vi "Error Query.vi"(8 "error in (no error)":errorcluster, 11 "VISA resource name":refnum<visa-resource-name>) -> (0 "error out":errorcluster, 1 "Error Message":string, 2 "Error Code (00)":i32, 3 "VISA resource name out":refnum<visa-resource-name>)   [LabVIEW 2015, in "Fluke 28x Series.lvlib"]
doc: "Queries the instrument for any errors in the instrument's error queue. It will continue to read errors until all errors have been read from the instrument. Any errors will be returned in the <B>error out</B> control.\n\n<B>Note:</B>\nThis VI is called automatically by most driver VIs so it is not usually necessary to call this in an application."
uses:
  <instrlib>/Fluke 28x Series/Fluke 28x Series.lvlib
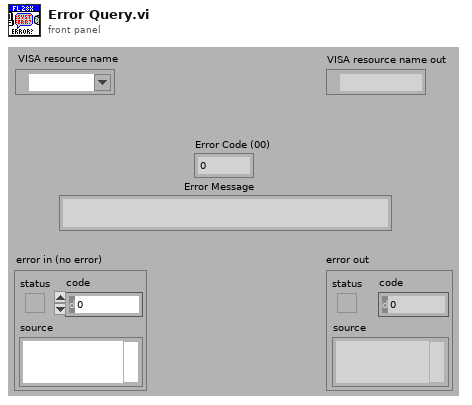
[diagram p1: front panel]
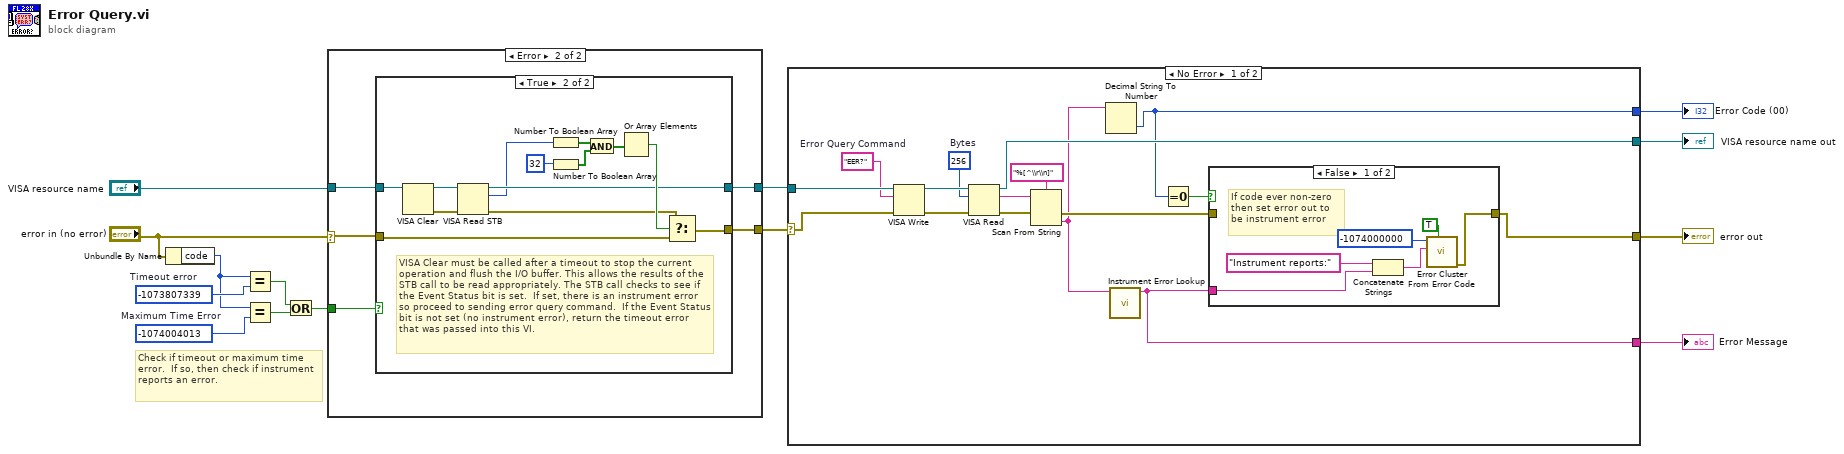
[diagram p0: block diagram]
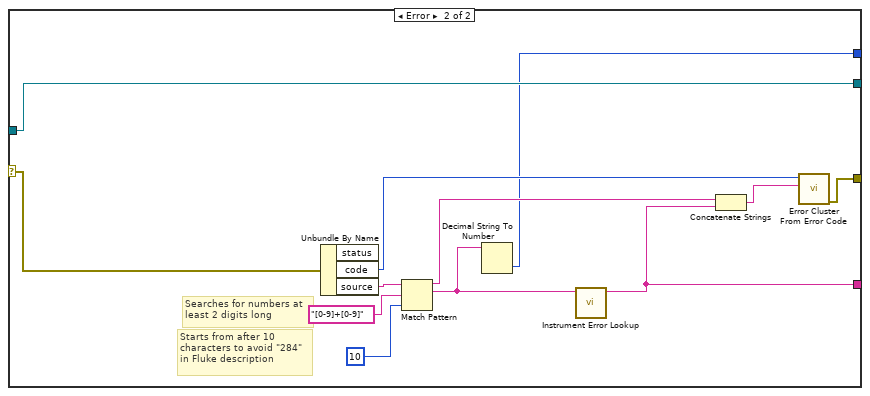
[diagram p5: hidden frame]
diagram:
  w6 = -1074004013  # Maximum Time Error
  w8 = -1073807339  # Timeout error
  # "Check if timeout or maximum time error.  If so, then check if instrument reports an error."
  n1 = Unbundle By Name("error in (no error)") -> ("code"=w7:i32)
  n2 = Equal?(x=w7, y=w8) -> (x = y?=w4:bool)
  n3 = Equal?(x=w7, y=w6) -> (x = y?=w5:bool)
  n4 = Or(x=w4, y=w5) -> (x .or. y?=w3:bool)
  n5 = case shown="Error" "error in (no error)" {
    selector: "error in (no error)" -> [w15 w19]
    tunnel: "VISA resource name" -> [w16 w21]
    tunnel: [w16 w20] -> w10
    tunnel: [w15 w18] -> w11
    tunnel: w3 -> [_ w17]
    frame No Error {
    }
    frame Error {
      n6 = case shown="True" w17 {
        tunnel: w21 -> [w23 w29]
        tunnel: [w23 w26] -> w20
        tunnel: w19 -> [w22 w32]
        tunnel: [w22 w31] -> w18
        frame False {
          # "Error code not a timeout, so best to pass on to user."
        }
        frame True {
          # "VISA Clear must be called after a timeout to stop the current operation and flush the I/O buffer. This allows the results of the  STB call to be read appropriately. The STB call checks to see if the Event Status bit is set.  If set, there is an instrument error so proceed to sending error query command.  If the Event Status bit is not set (no instrument error), return the timeout error that was passed into this VI."
          n7 = VISA Clear(VISA resource name=w29) -> (VISA resource name out=w28:refnum<visa-resource-name>, error out=w27:errorcluster)  [unwired: 1 in]
          n8 = VISA Read STB(8:w27, 11:w28) -> (0:w25:errorcluster, 2:w24:u16, 3:w26:refnum<visa-resource-name>)
          n9 = Number To Boolean Array(number=w24) -> (Boolean array=w33:bool[])
          n10 = Number To Boolean Array(number=32) -> (Boolean array=w35:bool[])
          n11 = And(x=w33, y=w35) -> (x .and. y?=w34:bool[])
          n12 = Or Array Elements(Boolean array=w34) -> (logical OR=w30:bool)
          n13 = Select(t=w25, s=w30, f=w32) -> (s? t:f=w31:errorcluster)
        }
      }
    }
  }
  n14 = case shown="No Error" w11 {
    selector: w11 -> [w50 w67]
    tunnel: [w52 w71] -> w14
    tunnel: w10 -> [w51 w71]
    tunnel: [w37 w64] -> w13
    tunnel: [w42 w62] -> w12
    tunnel: [w40 w60] -> w2
    frame No Error {
      w43 = "EER?"  # Error Query Command
      w48 = u32 256  # Bytes
      n15 = VISA Write(VISA resource name=w51, write buffer=w43, error in (no error)=w50) -> (VISA resource name out=w49:refnum<visa-resource-name>, error out=w47:errorcluster)  [unwired: 1 out]
      n16 = VISA Read(VISA resource name=w49, byte count=w48, error in (no error)=w47) -> (VISA resource name out=w52:refnum<visa-resource-name>, read buffer=w45:string, error out=w44:errorcluster)  [unwired: 1 out]
      n17 = Scan From String(format string="%[^\\r\\n]", input string=w45, error in=w44) -> (error out=w41:errorcluster, output 1=w38:string)  [unwired: 2 in, 2 out]
      n18 = Decimal String To Number(string=w38) -> (number=w40:i32)  [unwired: 2 in, 1 out]
      n19 = call <instrlib>:"Instrument Error Lookup.vi"("Error Code (00)"=w38) -> ("Error Message"=w42:string)  [unwired: 10 in]
      n20 = Equal To 0?(x=w40) -> (x = 0?=w39:bool)
      n21 = case shown="False" w39 {
        tunnel: [w54 w59] -> w37
        tunnel: w42 -> [w53 _]
        tunnel: w41 -> [_ w59]
        frame False {
          # "If code ever non-zero\nthen set error out to\nbe instrument error"
          n22 = Concatenate Strings("Instrument reports:" ("Source"), w53) -> (w55:string)
          n23 = call <vilib>:"Error Cluster From Error Code.vi"("show call chain? (False)"=TRUE, "error message (\"\")"=w55, "error code (0)"=-1074000000 ("Code")) -> ("error out"=w54:errorcluster)  [unwired: 6 in]
        }
        frame True {
        }
      }
    }
    frame Error {
      # "Starts from after 10\ncharacters to avoid \"284\"\nin Fluke description"
      # "Searches for numbers at\nleast 2 digits long"
      n24 = Unbundle By Name(w67) -> ("code"=w66:i32, "source"=w70:string)  [unwired: 1 out]
      n25 = Match Pattern(string=w70, regular expression="[0-9]+[0-9]", offset (0)=10) -> (before substring=w61:string, match substring=w65:string)  [unwired: 2 out]
      n26 = Decimal String To Number(string=w65) -> (number=w60:i32)  [unwired: 2 in, 1 out]
      n27 = call <instrlib>:"Instrument Error Lookup.vi"("Error Code (00)"=w65) -> ("Error Message"=w62:string)  [unwired: 10 in]
      n28 = Concatenate Strings(w61, w62) -> (w63:string)
      n29 = call <vilib>:"Error Cluster From Error Code.vi"("error message (\"\")"=w63, "error code (0)"=w66) -> ("error out"=w64:errorcluster)  [unwired: 7 in]
    }
  }
  "VISA resource name out" <- w14
  "error out" <- w13
  "Error Message" <- w12
  "Error Code (00)" <- w2
